vi "PING fpga子.vi"(11 "FPGA Reference Input":refnum<k21>) -> (2 "timed out?":bool, 3 "pulse width (uSec)":i32)   [LabVIEW 2017]
uses:
  <vilib>/robotics/Utilities/FPGA Utilities/Generate Digital Pulse (Ticks).vi
  <vilib>/rvi/eio/common/nirviEmuTemplateMethod_errors.vi
  <vilib>/robotics/Utilities/FPGA Utilities/Measure Digital Pulse Width (Ticks).vi
  <vilib>/eio/EIOMethodNode/EIOMethodNode.xnode
  <vilib>/eio/EIONode/EIONode.xnode
  <vilib>/robotics/Utilities/FPGA Utilities/NI_Robotics_FPGA Utilities.lvlib
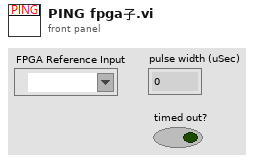
[diagram p1: front panel]
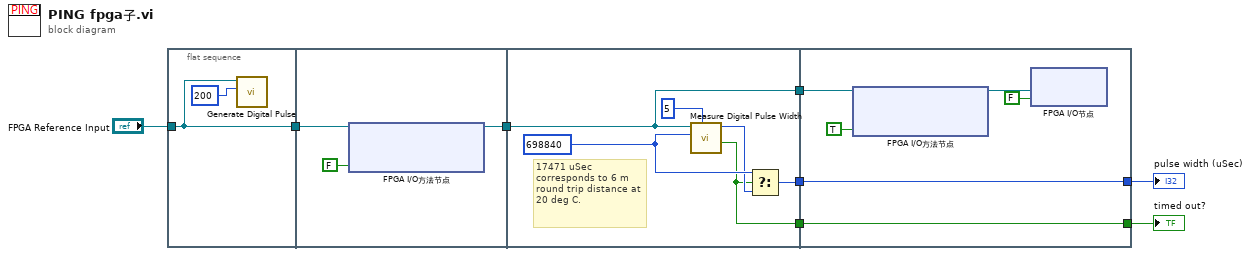
[diagram p0: block diagram]
diagram:
  n1 = flat-sequence {
    tunnel: [w9] -> w8
    tunnel: "FPGA Reference Input" -> [w9]
    tunnel: w8 -> [w12]
    tunnel: [w11] -> w7
    tunnel: w7 -> [w15]
    tunnel: [w19] -> w6
    tunnel: [w15] -> w5
    tunnel: [w16] -> w4
    tunnel: [w24] -> w2
    tunnel: [w25] -> w1
    tunnel: w6 -> [w25]
    tunnel: w5 -> [w20]
    tunnel: w4 -> [w24]
    frame #0 {
      n2 = call-poly <vilib>:"Generate Digital Pulse.vi"("pulse width (Ticks)"=u32 200 ("Count(uSec)"), "FPGA Reference Input"=w9) -> ()  [unwired: 10 in]
    }
    frame #1 {
      n3 = xnode "FPGA I/O方法节点"("FPGA I/O In"=w12, "Enable"=FALSE) -> ("FPGA I/O Out"=w11:refnum<k21>)
    }
    frame #2 {
      w18 = 698840 ("timeout (ticks)")
      # "17471 uSec corresponds to 6 m round trip distance at 20 deg C."
      n4 = call-poly <vilib>:"Measure Digital Pulse Width.vi"("cycles to filter (0)"=u16 5, "timeout (Ticks)"=w18, "FPGA Reference Input"=w15) -> ("timed out?"=w16:bool, "pulse width (Ticks)"=w17:i32)  [unwired: 7 in]
      n5 = Select(t=w18, s=w16, f=w17) -> (s? t:f=w19:i32)
    }
    frame #3 {
      n6 = xnode "FPGA I/O方法节点"("FPGA I/O In"=w20, "Enable"=TRUE) -> ("FPGA I/O Out"=w22:refnum<k21>)
      n7 = xnode "FPGA I/O节点"("I/O项"=FALSE ("I/O Item"), "FPGA I/O输入"=w22) -> ()  [unwired: 1 out]
    }
  }
  "timed out?" <- w2
  "pulse width (uSec)" <- w1
